vi "Read_Write_Trav_Config.vi"(1 "Traverse Name":string, 2 "Mode":T1(ring)) -> ()   [LabVIEW 2010]
uses:
  <vilib>/Instr/_visa.llb/VISA Find Search Mode.ctl
  Anemometry/Anemometry Sub Vis/Globals/Constants_global.vi
  Anemometry/Anemometry Sub Vis/Globals/Trav_pos_global.vi
  DriveConfigGlobal.vi
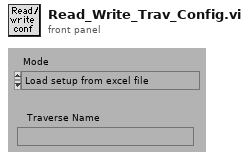
[diagram p1: front panel]
types:
  T1 = enum16{"Load setup from excel file", "Save setup to excel file"}
  T2 = typedef "DriveProperties.ctl" = cluster{"Channel Name":string, "Vel. Default":dbl, "Acc. Default":dbl, "Vel. Max":dbl, "Vel. Min":dbl, "Acc. Max":dbl, "Acc. Min":dbl, "Pulses/unit":dbl, "Address":u8, "Pulse Offset":i32, "Pos Tolerance":dbl, "Pulses/rev":dbl, "Backlash/Eng units":dbl, "Current Pos":dbl, "Ch Status":enum16{"Active", "Offline", "Simulate"}, "Port Name":string, "Axis Transform mode":string, "Metadata Ch Name":string, "Type":string}
  T3 = typedef "DriveStaticConfig.ctl" = cluster{"Correction Gain % (CG)":u16, "Dead Band (DB)":i32, "Dead Band Window (DW)":i32, "Encoder Resolution (ER)":i32, "Step Mode  (FSB)":u16, "Position Maintenance (FSC)":u16, "Stop on Stall (FSD)":u16, "Activate OP1 on stall (FSE)":u16, "Stop on Trigger 3 (FSF)":u16, "OP2 in Deadband (FSG)":u16, "Stall Detect (FSH)":u16, "Limit Disable (LD)":u16, "Motor Resolution (MR)":enum16{"200", "400", "1000", "2000", "4000", "5000", "10000", "12800", "18000", "20000", "21600", "25000", "25400", "25600", "36000", "50000", "278528", "425984", "507904", "614400", "655360", "819200", "1024000"}, "Limit Switch Sense (OSA)":u16, "Home Position (OSB)":u16, "Home Switch Sense (OSC)":u16, "Encoder Z for Home (OSD)":u16, "Reference edge of Home (OSH)":u16, "RS232 Echo Control (SSA)":u16, "Buffer at Limit (SSG)":u16, "Buffer at Stop (SSH)":u16, "Indexer Mode  (FSA)":u16, "Type":string, "ConfigString":string, "De Power Motor":enum16{"TRUE", "FALSE"}}
  T4 = cluster{"Channel Properties Out":T2, "Static Drive Configuration Out":T3}
  T5 = typedef "VISA Find Search Mode.ctl" = u32
  T6 = typedef "AxisConfigCluster.ctl" = cluster{"Channel Properties":T2, "Static Drive Configuration":T3}
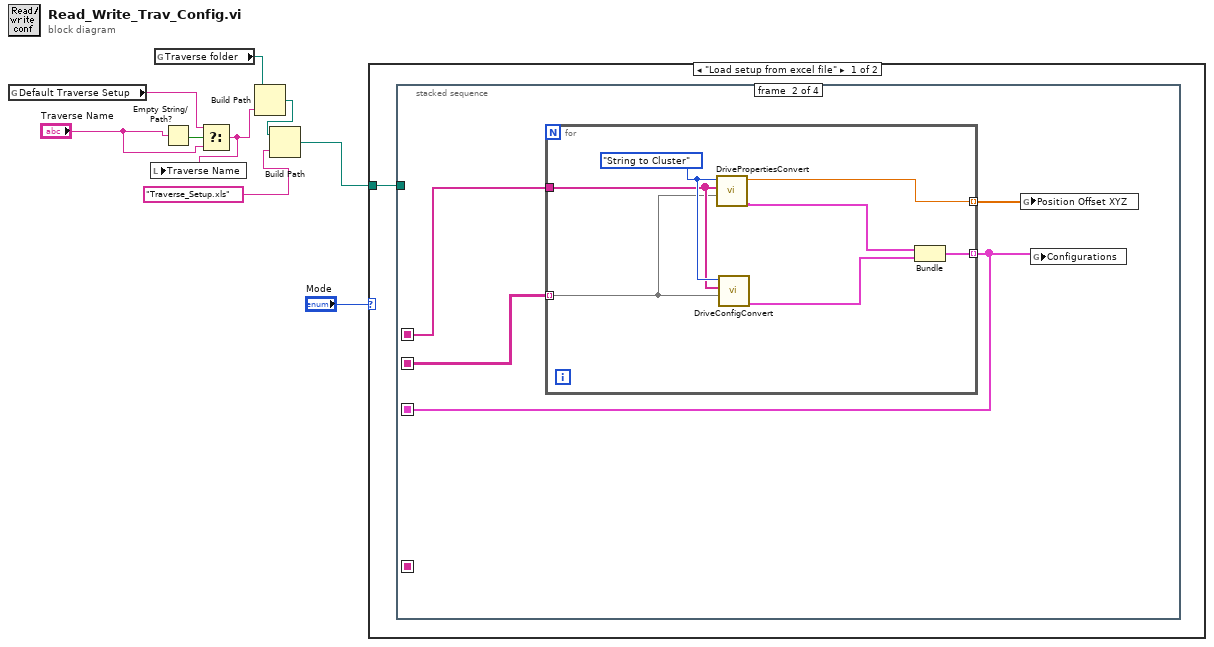
[diagram p0: block diagram]
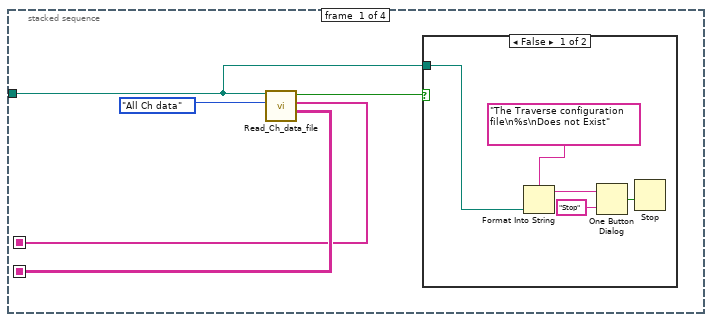
[diagram p2: hidden frame]
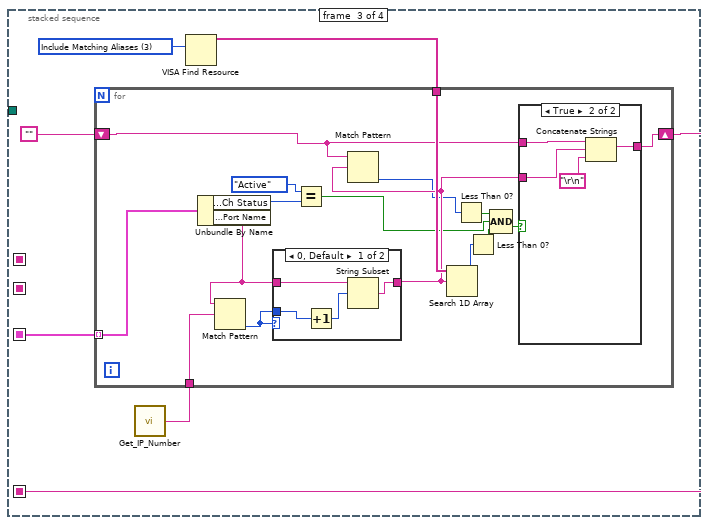
[diagram p4: hidden frame]
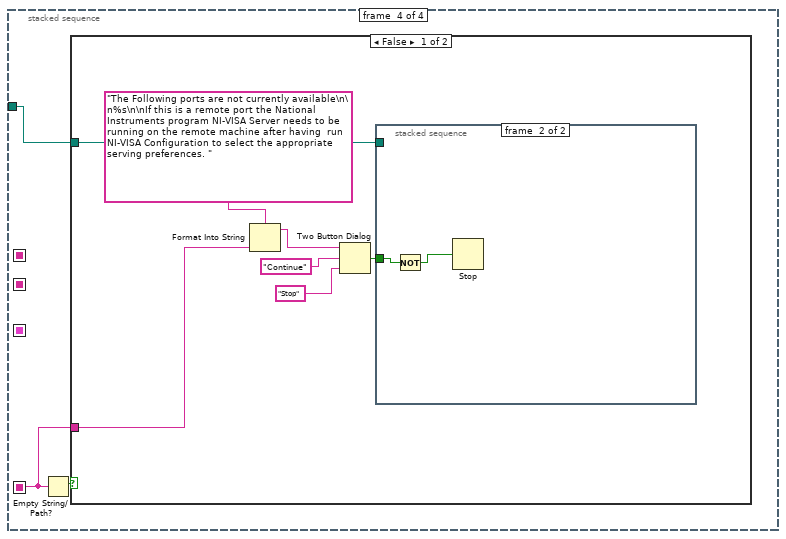
[diagram p7: hidden frame]
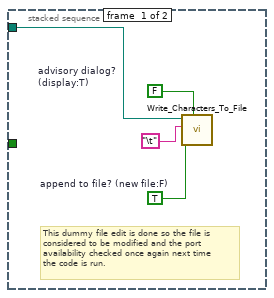
[diagram p8: hidden frame]
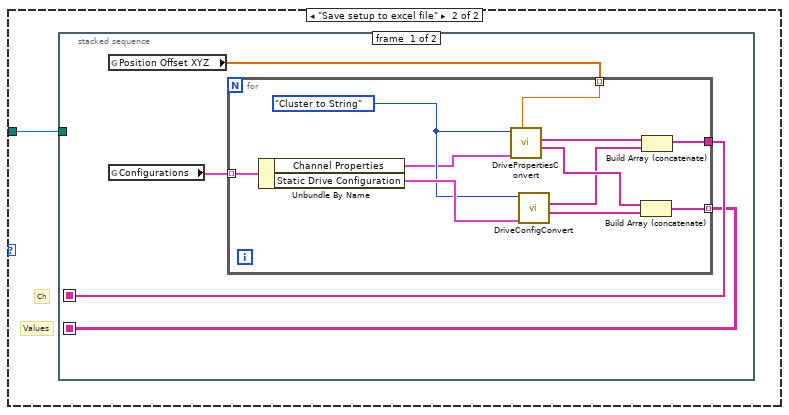
[diagram p10: hidden frame]
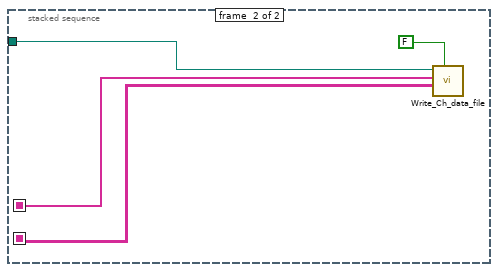
[diagram p11: hidden frame]
diagram:
  n1 = global read "Trav_pos_global.vi" "Default Traverse Setup"() -> (w4:string)
  n2 = global read "Constants_global.vi" "Traverse folder"() -> (w7:path)
  n3 = Empty String/Path?(string/path="Traverse Name") -> (empty?=w5:bool)
  n4 = Select(t=w4, s=w5, f="Traverse Name") -> (s? t:f=w1:string)
  n5 = local write "Traverse Name"(w1) -> ()
  n6 = Build Path(base path=w7, name or relative path=w1) -> (appended path=w6:path)
  n7 = Build Path(base path=w6, name or relative path="Traverse_Setup.xls" ("Substring")) -> (appended path=w8:path)
  n8 = case shown="\"Load setup from excel file\"" "Mode" {
    tunnel: w8 -> [w10 w80]
    frame "Load setup from excel file" {
      n9 = stacked-sequence {
        seq-local: [w14 _ _ _] -> [_ w23 _ _]
        seq-local: [w13 _ _ _] -> [_ w24 _ _]
        seq-local: [_ w22 _ _] -> [_ _ w36 _]
        seq-local: [_ _ w33 _] -> [_ _ _ w65]
        tunnel: w10 -> [w11 _ _ w64]
        frame #0 {
          n10 = call "Read_Ch_data_file.vi"("Output"=enum16{"All Ch data", "The last few rows"}."All Ch data", "Filename"=w11) -> ("Channel Values"=w14:string[][], "Merged Channels"=w13:string[], "exists?"=w12:bool)  [unwired: 3 in, 2 out]
          n11 = case shown="False" w12 {
            tunnel: w11 -> [w20 _]
            frame False {
              n12 = Format Into String(format string="The Traverse configuration file\n%s\nDoes not Exist" ("Format String"), w20) -> (resulting string=w18:string)  [unwired: 2 in, 1 out]
              n13 = One Button Dialog(message=w18, button name ("OK")="Stop") -> (true=w16:bool)
              n14 = Stop(stop? (T)=w16) -> ()
            }
            frame True {
            }
          }
        }
        frame #1 {
          n15 = for {
            tunnel: w24 -> [w30]
            tunnel: w23 -> [w29] mode=indexing
            tunnel: [w27] -> w22 mode=indexing
            tunnel: [w25] -> w21 mode=indexing
            w31 = enum16{"Cluster to String", "String to Cluster"}."String to Cluster" ("Mode")
            n16 = call "DrivePropertiesConvert.vi"("String in"=w29, "Ch names In"=w30, "Mode"=w31) -> ("Channel Properties Out"=w26:T2, "Position Offset Out"=w25:dbl)  [unwired: 2 in, 2 out]
            n17 = call "DriveConfigConvert.vi"("Values in"=w29, "Ch names In"=w30, "Mode"=w31) -> ("Static Drive Configuration Out"=w28:T3)  [unwired: 1 in, 3 out]
            n18 = Bundle("Channel Properties Out"=w26, "Static Drive Configuration Out"=w28) -> (w27:T4)  [unwired: 1 out]
          }
          n19 = global write "DriveConfigGlobal.vi" "Position Offset XYZ"(w21) -> ()
          n20 = global write "DriveConfigGlobal.vi" "Configurations"(w22) -> ()
        }
        frame #2 {
          w32 = T5 3 items=["Canonical Names Only"=0, "Aliases Only"=2, "Include Matching Aliases"=3, "Include All Aliases"=4] ("Search Mode")
          n21 = call "Get_IP_Number.vi"() -> ("IP Number"=w37:string)
          n22 = VISA Find Resource(10:w32) -> (3:w35:string[])  [unwired: 1 in, 3 out]
          n23 = for {
            tunnel: w37 -> [w53]
            tunnel: w36 -> [w51] mode=indexing
            tunnel: w35 -> [w49]
            shift-right: [w48] -> w33
            shift-left: "" -> [w47]
            n24 = Unbundle By Name(w51) -> ("Channel Properties Out.Ch Status"=w39:enum16{"Active", "Offline", "Simulate"}, "Channel Properties Out.Port Name"=w50:string)
            n25 = Match Pattern(string=w50, regular expression=w53) -> (offset past match=w52:i32)  [unwired: 4 out]
            n26 = case shown="0, Default" w52 {
              tunnel: [w59 w63] -> w46
              tunnel: w50 -> [w60 w63]
              tunnel: w52 -> [w62 _]
              frame 0, Default {
                n27 = Increment(x=w62) -> (x+1=w61:i32)
                n28 = String Subset(string=w60, offset (0)=w61) -> (substring=w59:string)  [unwired: 1 out]
              }
              frame -1 {
              }
            }
            n29 = Equal?(x=enum16{"Active", "Offline", "Simulate"}."Active" ("Channel Properties.Ch Status"), y=w39) -> (x = y?=w38:bool)
            n30 = Match Pattern(string=w47, regular expression=w46) -> (offset past match=w44:i32)  [unwired: 4 out]
            n31 = Search 1D Array(1D array=w49, element=w46) -> (index of element=w45:i32)  [unwired: 1 out]
            n32 = Less Than 0?(x=w44) -> (x < 0?=w41:bool)
            n33 = Less Than 0?(x=w45) -> (x < 0?=w43:bool)
            n34 = Compound Arithmetic op=AND(w41, w38, w43) -> (w42:bool)
            n35 = case shown="True" w42 {
              tunnel: w47 -> [w54 w58]
              tunnel: [w54 w57] -> w48
              tunnel: w46 -> [_ w56]
              frame False {
              }
              frame True {
                n36 = Concatenate Strings(w58, w56, "\r\n") -> (w57:string)
              }
            }
          }
        }
        frame #3 {
          n37 = Empty String/Path?(string/path=w65) -> (empty?=w66:bool)
          n38 = case shown="False" w66 {
            tunnel: w65 -> [w73 _]
            tunnel: w64 -> [w70 _]
            frame False {
              n39 = Format Into String(format string="The Following ports are not currently available\n\n%s\n\nIf this is a remote port the National Instruments program NI-VISA Server needs to be running on the remote machine after having  run NI-VISA Configuration to select the appropriate serving preferences. ", w73) -> (resulting string=w72:string)  [unwired: 2 in, 1 out]
              n40 = Two Button Dialog(message=w72, 1:"Stop" ("button name (\"OK\")"), 2:"Continue" ("T button name (\"OK\")")) -> (T button?=w69:bool)
              n41 = stacked-sequence {
                tunnel: w70 -> [w77 _]
                tunnel: w69 -> [_ w79]
                frame #0 {
                  w74 = FALSE  # advisory dialog? (display:T)
                  w75 = TRUE  # append to file? (new file:F)
                  # "This dummy file edit is done so the file is \nconsidered to be modified and the port \navailability checked once again next time\nthe code is run."
                  n42 = call "Write_Characters_To_File.vi"("file path (dialog if empty)"=w77, "advisory dialog? (display:T)"=w74, "character string"="\t", "append to file? (new file:F)"=w75) -> ()  [unwired: 1 in, 4 out]
                }
                frame #1 {
                  n43 = Not(x=w79) -> (.not. x?=w78:bool)
                  n44 = Stop(stop? (T)=w78) -> ()
                }
              }
            }
            frame True {
            }
          }
        }
      }
    }
    frame "Save setup to excel file" {
      # "Values"
      # "Ch"
      n45 = stacked-sequence {
        seq-local: [w84 _] -> [_ w98]
        seq-local: [w83 _] -> [_ w97]
        tunnel: w80 -> [_ w99]
        frame #0 {
          n46 = global read "DriveConfigGlobal.vi" "Position Offset XYZ"() -> (w81:dbl[])
          n47 = global read "DriveConfigGlobal.vi" "Configurations"() -> (w82:T6[])
          n48 = for {
            tunnel: w82 -> [w95] mode=indexing
            tunnel: [w88] -> w84
            tunnel: [w87] -> w83 mode=indexing
            tunnel: w81 -> [w85] mode=indexing
            w89 = enum16{"Cluster to String", "String to Cluster"}."Cluster to String" ("Mode")
            n49 = Unbundle By Name(w95) -> ("Channel Properties"=w86:T2, "Static Drive Configuration"=w94:T3)
            n50 = call "DrivePropertiesConvert.vi"("Position Offset In"=w85, "Channel Properties In"=w86, "Mode"=w89) -> ("String Values"=w93:string[], "Ch names"=w91:string[])  [unwired: 2 in, 2 out]
            n51 = call "DriveConfigConvert.vi"("Static Drive Configuration in"=w94, "Mode"=w89) -> ("String Values"=w92:string[], "Ch names"=w90:string[])  [unwired: 2 in, 2 out]
            n52 = Build Array (concatenate)(w93, w92) -> (w87:string[])
            n53 = Build Array (concatenate)(w91, w90) -> (w88:string[])
          }
        }
        frame #1 {
          n54 = call "Write_Ch_data_file.vi"("exists?"=FALSE, "Channel Values"=w97, "Channel names"=w98, "Filename"=w99) -> ()  [unwired: 4 in, 4 out]
        }
      }
    }
  }
